vi "Send User Event.vi"(8 "error in (no error)":errorcluster caption="에러 입력(에러 없음)", 10 "Event":cluster{"Key":string, "Command":string}, 11 "User Event in":refnum<user-event>) -> (0 "error out":errorcluster caption="에러 출력", 3 "User Event out":refnum<user-event>)   [LabVIEW 2018, in "User Event.lvlib"]
uses:
  User Event.lvlib
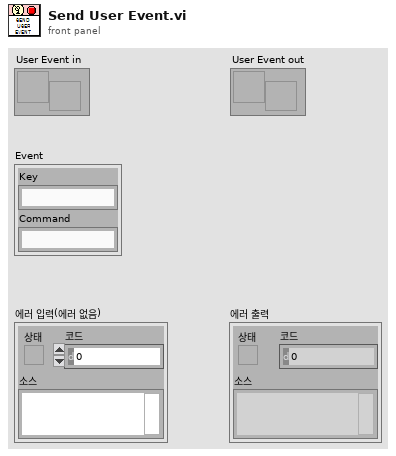
[diagram p1: front panel]
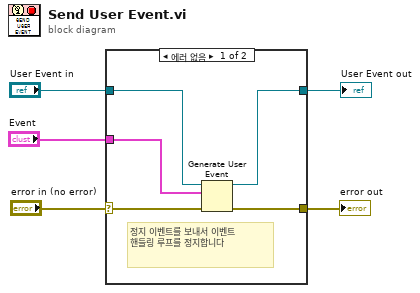
[diagram p0: block diagram]
diagram:
  n1 = case shown="에러 없음" "error in (no error)" {
    selector: "error in (no error)" -> [w8 w12]
    tunnel: [w10 w12] -> w5
    tunnel: "User Event in" -> [w9 w11]
    tunnel: "Event" -> [w7 _]
    tunnel: [w6 w11] -> w1
    frame No Error {
      # "정지 이벤트를 보내서 이벤트 핸들링 루프를 정지합니다"
      n2 = Generate User Event(user event=w9, event data cluster=w7, error in=w8) -> (user event out=w6:refnum<user-event>, error out=w10:errorcluster)  [unwired: 1 in]
    }
    frame Error {
    }
  }
  "error out" <- w5
  "User Event out" <- w1
